vi "Get Keypad Value(LV2015).vi"(8 "error in (no error)":errorcluster, 11 "Expect VK Value":i32(ring)=13 items=["Enter"=13, "Space"=32, "Delete"=46]) -> (0 "error out":errorcluster, 1 "Key State":i16, 2 "Target VK Value":i32, 3 "Result":bool, 5 "VK List":u8[](array[numeric]))   [LabVIEW 2015]
uses:
  user32.dll
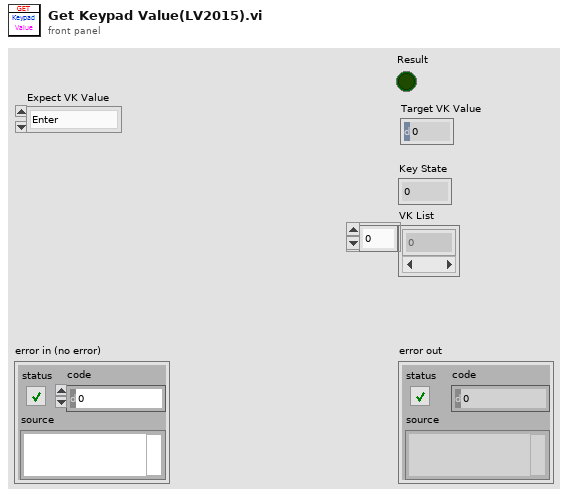
[diagram p1: front panel]
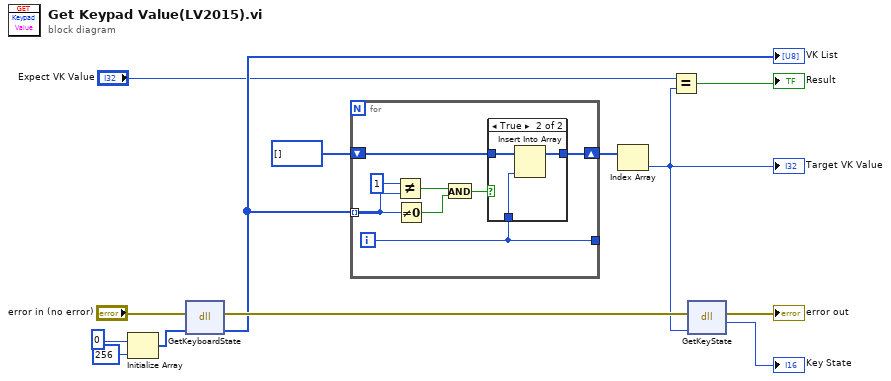
[diagram p0: block diagram]
diagram:
  n1 = Initialize Array(u8 0 ("arg1"), 256 ("dimension size")) -> (w11:u8[])
  n2 = dll-call lib="user32.dll" fn="GetKeyboardState"(error in="error in (no error)", "vk"=w11) -> (error out=w10:errorcluster, "vk"=w8:u8[])  [unwired: 3 in, 1 out]
  "VK List" <- w8
  n3 = for {
    tunnel: w8 -> [w21] mode=indexing
    tunnel: [w14] -> _
    shift-right: [w15] -> w6
    shift-left: i32[] [] ("VK Value List") -> [w16]
    i -> [w14]
    n4 = Not Equal?(x=u8 1, y=w21) -> (x != y?=w19:bool)
    n5 = Not Equal To 0?(x=w21) -> (x != 0?=w18:bool)
    n6 = And(x=w19, y=w18) -> (x .and. y?=w17:bool)
    n7 = case shown="True" w17 {
      tunnel: w16 -> [w22 w25]
      tunnel: [w22 w24] -> w15
      tunnel: w14 -> [_ w23]
      frame False {
      }
      frame True {
        n8 = Insert Into Array(array=w25, new element=w23) -> (w24:i32[])  [unwired: 1 in]
      }
    }
  }
  n9 = Index Array(array=w6) -> (element=w2:i32)  [unwired: 1 in]
  "Target VK Value" <- w2
  n10 = Equal?(x="Expect VK Value", y=w2) -> (x = y?=→"Result":bool)
  n11 = dll-call lib="user32.dll" fn="GetKeyState"(error in=w10, "vk"=w2) -> (error out=→"error out":errorcluster, "return type"=→"Key State":i16)  [unwired: 3 in, 1 out]
